vi "Data logging.vi"(9 "Array 2":T3(array[cluster]), 10 "Array":string[](array[string]), 11 "Array 3":T2(array[cluster])) -> (2 "Data logged":string[][](array[string]), 3 "Logging FIle Path":path)   [LabVIEW 2021]
uses:
  Type defs/Current moisteure level.ctl
  <vilib>/Utility/file.llb/Write Delimited Spreadsheet (string).vi
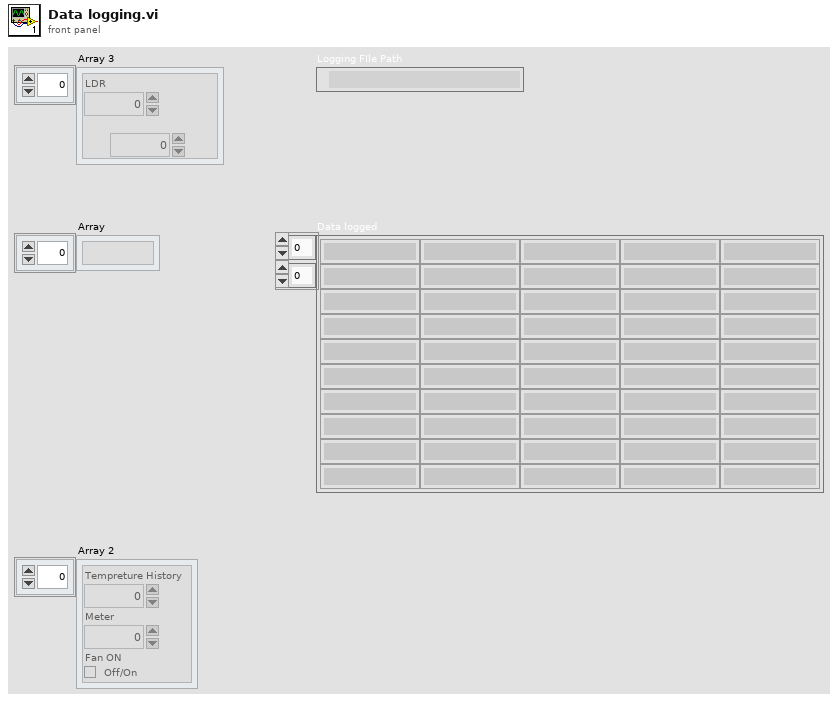
[diagram p1: front panel]
types:
  T1 = typedef "Current moisteure level.ctl" = u32
  T2 = cluster{"LDR":u32, "Current Moisture Level":T1}[]
  T3 = cluster{"Tempreture History":i32, "Meter":u32, "Fan ON":bool}[]
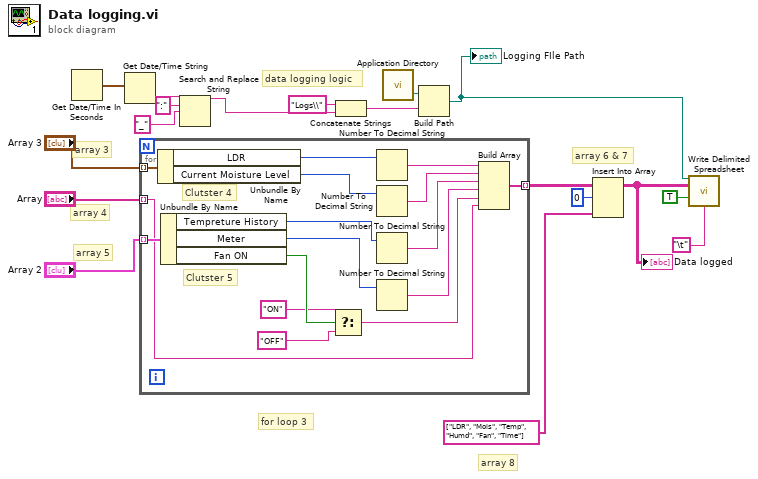
[diagram p0: block diagram]
diagram:
  # "data logging logic"
  # "for loop 3"
  # "array 8"
  # "array 6 & 7"
  # "array 5"
  # "array 4"
  # "array 3"
  n1 = Get Date/Time In Seconds() -> (seconds since 1Jan1904=w5:timestamp)
  n2 = Get Date/Time String(seconds (now)=w5) -> (time string=w6:string)  [unwired: 2 in, 1 out]
  n3 = for {
    tunnel: "Array 3" -> [w34] mode=indexing
    tunnel: "Array 2" -> [w33] mode=indexing
    tunnel: "Array" -> [w20] mode=indexing
    tunnel: [w19] -> w11 mode=indexing
    # "Clutster 5"
    # "Clutster 4"
    n4 = Unbundle By Name(w34) -> ("LDR"=w32:u32, "Current Moisture Level"=w31:T1)
    n5 = Unbundle By Name(w33) -> ("Tempreture History"=w30:i32, "Meter"=w29:u32, "Fan ON"=w28:bool)
    n6 = Select(t="ON" ("time string"), s=w28, f="OFF" ("time string")) -> (s? t:f=w21:string)
    n7 = Number To Decimal String(number=w32) -> (decimal integer string=w25:string)  [unwired: 1 in]
    n8 = Number To Decimal String(number=w31) -> (decimal integer string=w24:string)  [unwired: 1 in]
    n9 = Number To Decimal String(number=w30) -> (decimal integer string=w23:string)  [unwired: 1 in]
    n10 = Number To Decimal String(number=w29) -> (decimal integer string=w22:string)  [unwired: 1 in]
    n11 = Build Array(w25, w24, w23, w22, w21, w20) -> (w19:string[])
  }
  n12 = Search and Replace String(input string=w6, search string=":", replace string="_" ("replace string (\"\")")) -> (result string=w17:string)  [unwired: 5 in, 3 out]
  n13 = Concatenate Strings("Logs\\" ("string"), w17) -> (w18:string)
  n14 = call <vilib>:"Application Directory.vi"() -> ("Application Directory"=w4:path)
  n15 = Build Path(base path=w4, name or relative path=w18) -> (appended path=w9:path)
  "Logging FIle Path" <- w9
  n16 = Insert Into Array(array=w11, index (row)=0, new element=string[] ["LDR", "Mois", "Temp", "Humd", "Fan", "Time"] ("new element/subarray")) -> (w15:string[][])  [unwired: 1 in]
  "Data logged" <- w15
  n17 = call-poly <vilib>:"Write Delimited Spreadsheet.vi"("file path (dialog if empty)"=w9, "2D data"=w15, "append to file? (new file:F)"=TRUE, "delimiter (\\t)"="\t") -> ()  [unwired: 10 in, 2 out]
